vi "loadControlsFromTarget.vi"(8 "error in (no error)":errorcluster, 9 "ConnectionData":T1, 10 "ControlsToLoad":refnum<vi>[](array[refnum]), 11 "ConfigXMLControls":T2) -> (0 "error out":errorcluster)   [LabVIEW 2015]
uses:
  ConfigXMLControl.ctl
  General/RemoteFiles/connectionData.ctl
  <vilib>/NI/GXML/_subVIs/GXML SearchParser/Search Parser.vi
  <vilib>/NI/GXML/GXML.lvlib
panel:
  # "Fetches the current file from the target, saves it to temp"
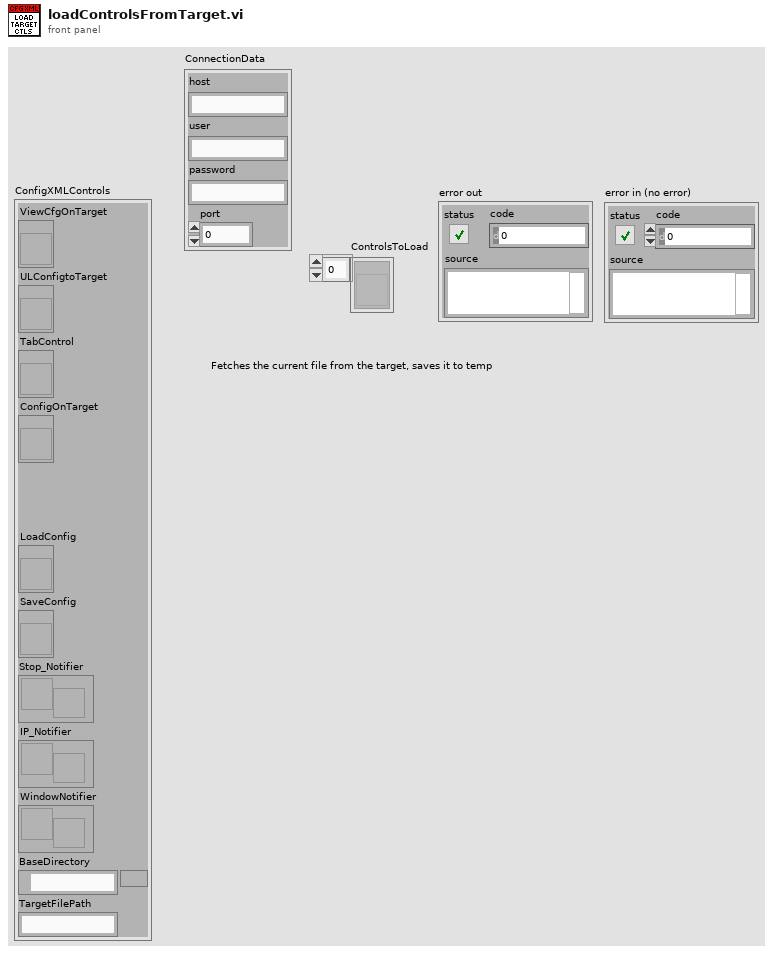
[diagram p1: front panel]
types:
  T1 = typedef "connectionData.ctl" = cluster{"host":string, "user":string, "password":string, "port":u16}
  T2 = typedef "ConfigXMLControl.ctl" = cluster{"ViewCfgOnTarget":refnum<vi>, "ULConfigtoTarget":refnum<vi>, "TabControl":refnum<vi>, "ConfigOnTarget":refnum<vi>, "LoadConfig":refnum<vi>, "SaveConfig":refnum<vi>, "Stop_Notifier":refnum<notifier>, "IP_Notifier":refnum<notifier>, "WindowNotifier":refnum<notifier>, "BaseDirectory":path, "TargetFilePath":string}
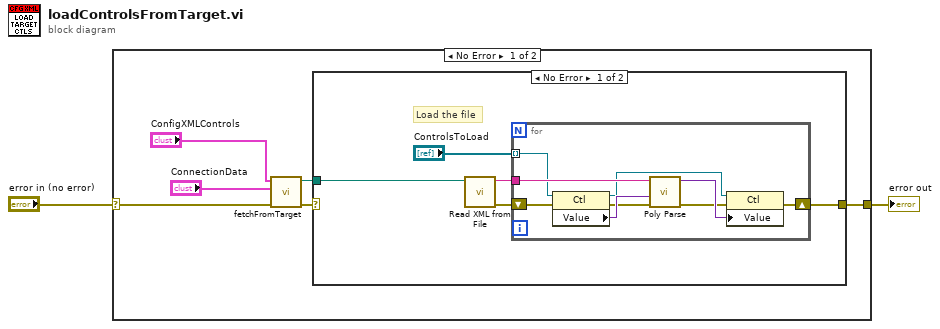
[diagram p0: block diagram]
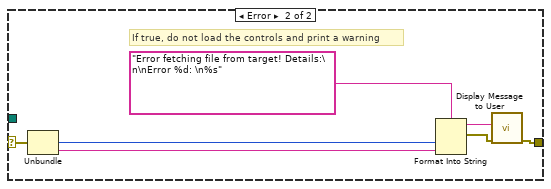
[diagram p2: hidden frame]
diagram:
  n1 = case shown="No Error" "error in (no error)" {
    selector: "error in (no error)" -> [w3 w30]
    tunnel: [w8 w30] -> w2
    frame No Error {
      n2 = call "fetchFromTarget.vi"("error in (no error)"=w3, "ConnectionData"="ConnectionData", "ConfigXMLControls"="ConfigXMLControls") -> ("error out"=w6:errorcluster, "path out"=w5:path)  [unwired: 5 in, 2 out]
      n3 = case shown="No Error" w6 {
        selector: w6 -> [_ w29]
        tunnel: [w11 w23] -> w8
        tunnel: w5 -> [w10 _]
        frame No Error {
          # "Load the file"
          n4 = call <vilib>:"Read XML from File.vi"("XML File Path"=w10) -> ("error out"=w12:errorcluster, "XML String Out"=w13:string)  [unwired: 9 in]
          n5 = for {
            tunnel: w13 -> [w22]
            tunnel: "ControlsToLoad" -> [w21] mode=indexing
            shift-right: [w14] -> w11
            shift-left: w12 -> [w15]
            n6 = property class="Ctl"(reference=w21, error in=w15) -> (reference out=w18:refnum<vi>, error out=w17:errorcluster, "Value"=w20:variant)
            n7 = call-poly <vilib>:"Poly Parse.vi"("error in"=w17, "TypeDesc"=w20, "XML String In"=w22) -> ("error out"=w16:errorcluster, "Parsed Data"=w19:variant)  [unwired: 7 in]
            n8 = property class="Ctl"(reference=w18, error in=w16, "Value"=w19) -> (error out=w14:errorcluster)  [unwired: 1 out]
          }
        }
        frame Error {
          # "If true, do not load the controls and print a warning"
          n9 = Unbundle(w29) -> ("code"=w28:i32, "source"=w27:string)  [unwired: 1 out]
          n10 = Format Into String(format string="Error fetching file from target! Details:\n\nError %d: \n%s" ("Message"), w28, w27) -> (resulting string=w25:string, error out=w24:errorcluster)  [unwired: 2 in]
          n11 = call "Display Message to User"("error in (no error)"=w24, "Message"=w25) -> ("error out"=w23:errorcluster)  [unwired: 8 in, 1 out]
        }
      }
    }
    frame Error {
    }
  }
  "error out" <- w2
